vi "InitTimeOfFlightSensors.vi"(8 "error in (no error)":errorcluster, 11 "LINX Resource":T2) -> (0 "error out":errorcluster, 2 "VL6180 Resources":T1[](array[typedef]) {"I2C Slave Address" format="%02x"}, 3 "LINX Resource Out":T2)   [LabVIEW 2014]
uses:
  <vilib>/MakerHub/LINX/LMH-LINX.lvlib
  <vilib>/MakerHub/LINX/Public/Peripherals/Digital/Digital Write 1 Chan.vi
  <vilib>/MakerHub/LINX/Private/Type Defs/Platform.ctl
  <vilib>/MakerHub/LINX/Private/Type Defs/Interface.ctl
  <vilib>/MakerHub/LINX/Private/Device/Type Defs/TCP Config.ctl
  <vilib>/MakerHub/LINX/Private/Device/Device.lvlib
  <vilib>/MakerHub/LINX/Private/Device/Type Defs/Channels.ctl
  <vilib>/MakerHub/LINX/Private/Device/Type Defs/LINX Device Config.ctl
  <vilib>/MakerHub/LINX/Private/Type Defs/LINX Ref.ctl
  Sensors/Time of Flight - VL6180/VL6180 Resource.ctl
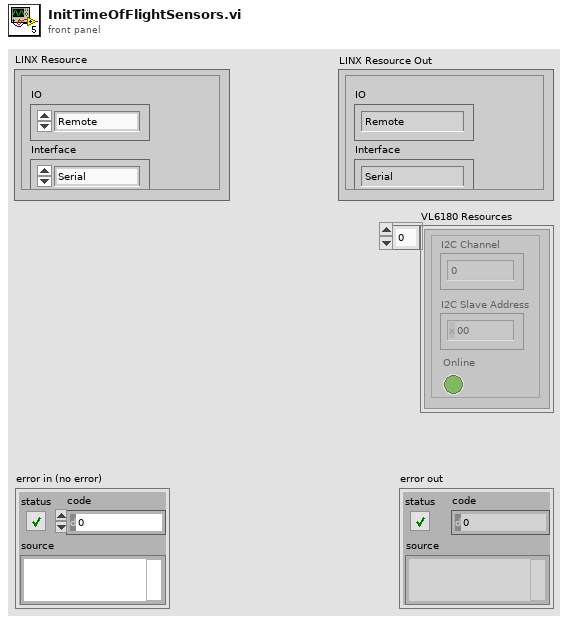
[diagram p1: front panel]
types:
  T1 = typedef "VL6180 Resource.ctl" = cluster{"I2C Channel":u8, "I2C Slave Address":u8, "Online":bool}
  T2 = typedef "LMH-LINX.lvlib/LINX Ref.ctl" = cluster{"IO":T3, "Interface":T4, "LINX Device Config":T5}
  T3 = typedef "LMH-LINX.lvlib/Platform.ctl" = enum16{"Remote", "Local"}
  T4 = typedef "LMH-LINX.lvlib/Interface.ctl" = enum16{"Serial", "TCP"}
  T5 = typedef "LMH-LINX.lvlib/Device.lvlib/LINX Device Config.ctl" = cluster{"Interface":T4, "COM Port":refnum<visa-resource-name>, "TCP Configuration":T6, "Device Family":u8, "Device ID":u8, "Device Name":string, "TCP Ref":refnum<k5>, "Channels":T7}
  T6 = typedef "LMH-LINX.lvlib/Device.lvlib/TCP Config.ctl" = cluster{"IP Address":string, "Port":u16}
  T7 = typedef "LMH-LINX.lvlib/Channels.ctl" = cluster{"DI":u8[], "DO":u8[], "AI":u8[], "AO":u8[], "PWM":u8[], "QE":u8[], "UART":u8[], "I2C 2":u8[], "SPI":u8[], "CAN":u8[], "Servo":u8[], "AI Ref (V)":dbl, "AI Resolution (Bits)":u8, "AO Ref (V)":dbl, "AO Resolution (Bits)":u8}
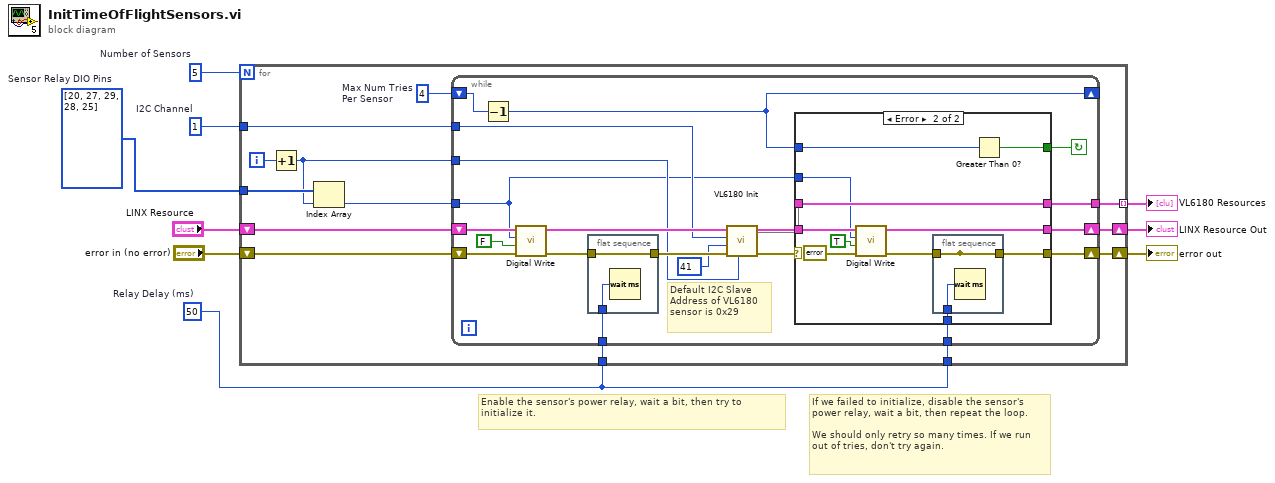
[diagram p0: block diagram]
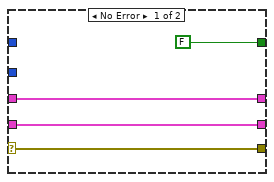
[diagram p2: hidden frame]
diagram:
  w3 = u32 50  # Relay Delay (ms)
  w6 = u8[] [20, 27, 29, 28, 25]  # Sensor Relay DIO Pins
  w8 = u8 1  # I2C Channel
  w9 = 5  # Number of Sensors
  # "If we failed to initialize, disable the sensor's power relay, wait a bit, then repeat the loop.\n\nWe should only retry so many times. If we run out of tries, don't try again."
  # "Enable the sensor's power relay, wait a bit, then try to initialize it."
  n1 = for {
    N: w9 -> [_]
    tunnel: w8 -> [w16]
    tunnel: w6 -> [w21]
    shift-right: [w13] -> w5
    shift-left: "error in (no error)" -> [w19]
    shift-right: [w12] -> w2
    shift-left: "LINX Resource" -> [w18]
    tunnel: w3 -> [w17]
    tunnel: w3 -> [w14]
    tunnel: [w11] -> w1 mode=indexing
    i -> [w22]
    w10 = 4  # Max Num Tries Per Sensor
    n2 = Increment(x=w22) -> (x+1=w15:i32)
    n3 = Index Array(array=w21, index=w15) -> (element=w20:u8)
    n4 = while {
      tunnel: w20 -> [w23]
      shift-right: [w30] -> w12
      shift-left: w18 -> [w43]
      shift-right: [w29] -> w13
      shift-left: w19 -> [w42]
      tunnel: w17 -> [w39]
      tunnel: w16 -> [w34]
      tunnel: w15 -> [w36]
      tunnel: w14 -> [w31]
      tunnel: [w27] -> w11
      shift-right: [w24] -> _
      shift-left: w10 -> [w26]
      stop <- w25 continue-if-true
      # "Default I2C Slave Address of VL6180 sensor is 0x29"
      n5 = Decrement(x=w26) -> (x-1=w24:i32)
      n6 = call-poly <vilib>:"Digital Write.vi"("Error In"=w42, "Output Value"=FALSE, "DO Channel"=w23, "LINX Resource"=w43) -> ("Error Out"=w40:errorcluster, "LINX Resource"=w37:T2)  [unwired: 6 in]
      n7 = flat-sequence {
        tunnel: [w62] -> w38
        tunnel: w40 -> [w62]
        tunnel: w39 -> [w61]
        frame #0 {
          n8 = Wait (ms)(milliseconds to wait=w61) -> ()  [unwired: 1 out]
        }
      }
      n9 = call "VL6180 Init.vi"("Change Slave Address"=w36, "Error In"=w38, "I2C Slave Address"=u8 41 ("I2C Slave Address (0)"), "I2C Channel"=w34, "LINX Resource"=w37) -> ("Error Out"=w33:errorcluster, "LINX Resource"=w32:T2, 5:w28)  [unwired: 3 in, 1 out]
      n10 = case shown="Error" w33 {
        selector: w33 -> [w46 _]
        tunnel: w32 -> [w47 w58]
        tunnel: w31 -> [_ w56]
        tunnel: [w47 w55] -> w30
        tunnel: [w46 w54] -> w29
        tunnel: w28 -> [w45 w52]
        tunnel: [w45 w52] -> w27
        tunnel: [FALSE w51] -> w25
        tunnel: w24 -> [_ w50]
        tunnel: w23 -> [_ w49]
        frame No Error {
        }
        frame Error {
          n11 = call-poly <vilib>:"Digital Write.vi"("Error In"=errorcluster {"status"=FALSE, "code"=0, "source"=""}, "Output Value"=TRUE, "DO Channel"=w49, "LINX Resource"=w58) -> ("Error Out"=w57:errorcluster, "LINX Resource"=w55:T2)  [unwired: 6 in]
          n12 = flat-sequence {
            tunnel: [w59] -> w54
            tunnel: [w59] -> _
            tunnel: w56 -> [w60]
            tunnel: w57 -> [w59]
            frame #0 {
              n13 = Wait (ms)(milliseconds to wait=w60) -> ()  [unwired: 1 out]
            }
          }
          n14 = Greater Than 0?(x=w50) -> (x > 0?=w51:bool)
        }
      }
    }
  }
  "error out" <- w5
  "LINX Resource Out" <- w2
  "VL6180 Resources" <- w1
